vi "My Circ Buff Init.vi"(8 "error in":errorcluster, 11 "circular buffer info":T1={"buff ref1"=refnum, "buff ref2"=refnum, "buffer1 path"=path "C:/perforce/users/CraigClaassen/content/CircBuff/buffer/buff1.buf", "buffer2 path"=path "C:/perforce/users/CraigClaassen/content/CircBuff/buffer/buff2.buf", "archive directory"=path "", "xml header"="", "num blocks  prior"=0, "num blocks after"=0, "blocks/event"=0, "samples/block"=0, "bytes/sample"=0, "number of channels"=2, "samples/block/channel"=10000, "read buffer ref queue"=refnum, "Event delay queue"=refnum, "command queue"=refnum}) -> (0 "error out":errorcluster, 3 "circular buffer info out":T1={"buff ref1"=refnum, "buff ref2"=refnum, "buffer1 path"=path "C:/perforce/users/CraigClaassen/content/CircBuff/buffer/buff1.buf", "buffer2 path"=path "C:/perforce/users/CraigClaassen/content/CircBuff/buffer/buff2.buf", "archive directory"=path "", "xml header"="", "num blocks  prior"=0, "num blocks after"=0, "blocks/event"=0, "samples/block"=0, "bytes/sample"=0, "number of channels"=2, "samples/block/channel"=10000, "read buffer ref queue"=refnum, "Event delay queue"=refnum, "command queue"=refnum})   [LabVIEW 2013]
uses:
  My circular buffer info.ctl
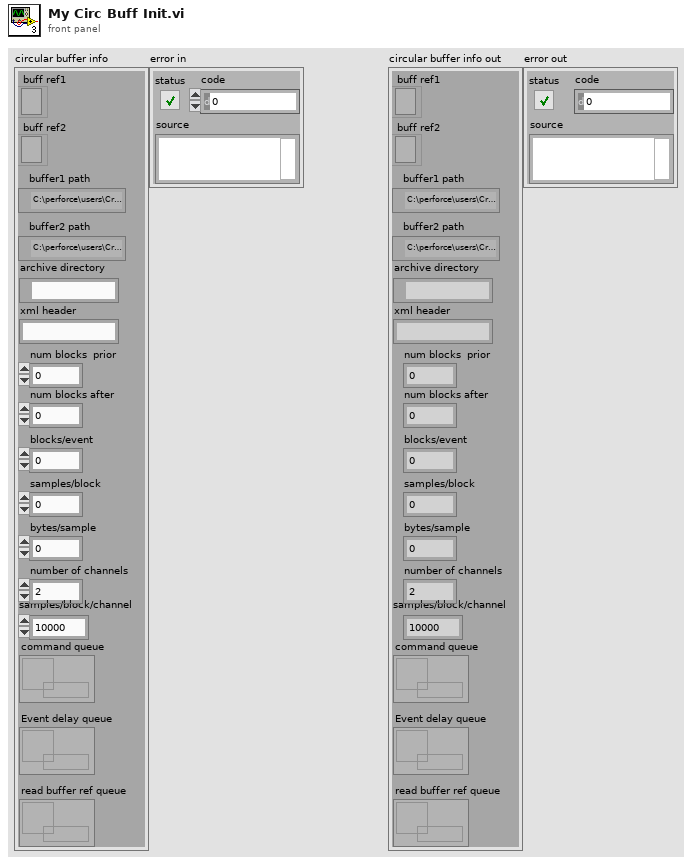
[diagram p1: front panel]
types:
  T1 = typedef "My circular buffer info.ctl" = cluster{"buff ref1":refnum<file>, "buff ref2":refnum<file>, "buffer1 path":path, "buffer2 path":path, "archive directory":path, "xml header":string, "num blocks  prior":i32, "num blocks after":i32, "blocks/event":i32, "samples/block":i32, "bytes/sample":i32, "number of channels":i32, "samples/block/channel":i32, "read buffer ref queue":refnum<queue>, "Event delay queue":refnum<queue>, "command queue":refnum<queue>}
  T2 = cluster{"filename":string, "bytes to write":i32, "archive mode":enum16{"direct", "append"}}
  T3 = cluster{"number of channels":i32, "samples/block/channel":i32, "bytes/sample":i32}
  T4 = enum16{"open", "replace", "create", "open or create", "replace or create", "replace or create with confirmation"}
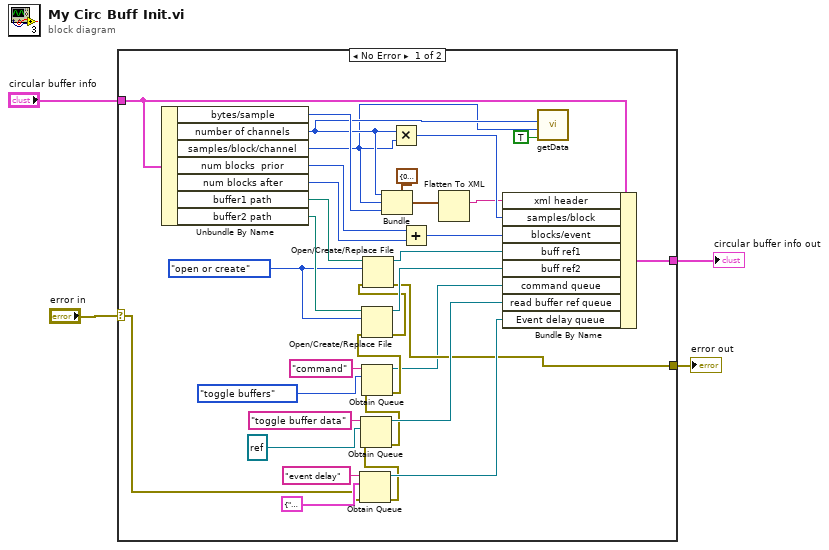
[diagram p0: block diagram]
diagram:
  n1 = case shown="No Error" "error in" {
    selector: "error in" -> [w14 w38]
    tunnel: "circular buffer info" -> [w16 w39]
    tunnel: [w15 w39] -> w2
    tunnel: [w9 w38] -> w1
    frame No Error {
      w26 = T4."open or create" ("operation (0:open)")
      n2 = Unbundle By Name(w16) -> ("bytes/sample"=w35:i32, "number of channels"=w8:i32, "samples/block/channel"=w7:i32, "num blocks  prior"=w32:i32, "num blocks after"=w31:i32, "buffer1 path"=w28:path, "buffer2 path"=w27:path)
      n3 = Obtain Queue(name (unnamed)="event delay", element data type=T2 {"filename"="", "bytes to write"=0, "archive mode"=enum."direct"} ("Event delay info"), error in (no error)=w14) -> (queue out=w19:refnum<queue>, error out=w13:errorcluster)  [unwired: 2 in, 1 out]
      n4 = Obtain Queue(name (unnamed)="toggle buffer data", element data type=refnum<file> refnum ("Byte Stream File Refnum"), error in (no error)=w13) -> (queue out=w20:refnum<queue>, error out=w12:errorcluster)  [unwired: 2 in, 1 out]
      n5 = Obtain Queue(name (unnamed)="command", element data type=enum16{"toggle buffers", "data event", "stop"}."toggle buffers" ("cmd enum"), error in (no error)=w12) -> (queue out=w5:refnum<queue>, error out=w11:errorcluster)  [unwired: 2 in, 1 out]
      n6 = Open/Create/Replace File(file path (use dialog)=w27, error in=w11, operation (0:open)=w26) -> (refnum out=w25:refnum<file>, error out=w10:errorcluster)  [unwired: 3 in, 1 out]
      n7 = Open/Create/Replace File(file path (use dialog)=w28, error in=w10, operation (0:open)=w26) -> (refnum out=w29:refnum<file>, error out=w9:errorcluster)  [unwired: 3 in, 1 out]
      n8 = Bundle(cluster=T3 {"number of channels"=0, "samples/block/channel"=0, "bytes/sample"=0} ("My data config"), "number of channels"=w8, "samples/block/channel"=w7, "bytes/sample"=w35) -> (w34:T3)
      n9 = Multiply(x=w8, y=w7) -> (x*y=w37:i32)
      n10 = Add(x=w32, y=w31) -> (x+y=w30:i32)
      n11 = Flatten To XML(anything=w34) -> (xml string=w33:string)
      n12 = Bundle By Name(cluster=w16, "xml header"=w33, "samples/block"=w37, "blocks/event"=w30, "buff ref1"=w29, "buff ref2"=w25, "command queue"=w5, "read buffer ref queue"=w20, "Event delay queue"=w19) -> (w15:T1)
      n13 = call "getData.vi"("Init (F)"=TRUE, "samples/block/channel"=w7, "number of channels"=w8) -> ()  [unwired: 4 in, 1 out]
    }
    frame Error {
    }
  }
  "circular buffer info out" <- w2
  "error out" <- w1
